vi "Set Fill Mode.vi"(8 "error in (no error)":errorcluster, 10 "Fill Mode":T1="ON", 11 "Instrument.1820 in":refnum<class "Instrument.Oxford1820.lvclass">) -> (0 "error out":errorcluster, 2 "Response":string, 3 "Instrument.1820 in":refnum<class "Instrument.Oxford1820.lvclass">)   [LabVIEW 2016, in "Instrument.Oxford1820.lvclass"]
uses:
  Instrument.Oxford1820.lvclass
  Typedefs/Fill Mode-Combo.ctl
  Typedefs/Instrument.Oxford1820.Commands-enum.ctl
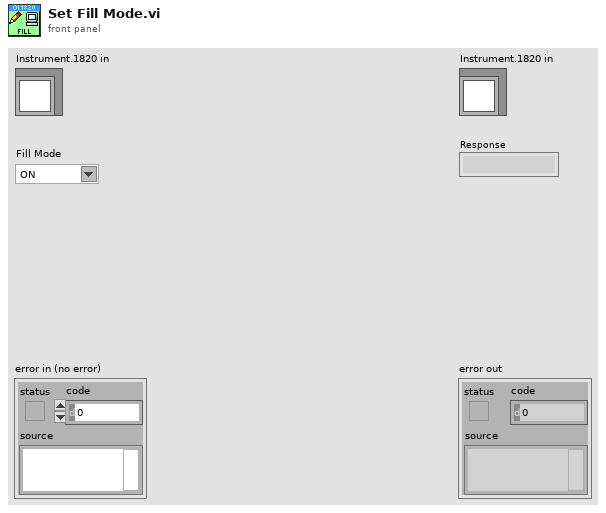
[diagram p1: front panel]
types:
  T1 = typedef "Instrument.Oxford1820.lvclass/Fill Mode-Combo.ctl" = string
  T2 = typedef "Instrument.Oxford1820.lvclass/Instrument.Oxford1820.Commands-enum.ctl" = enum16{"setAction", "setTarget", "setSwitchHeat", "setLambda", "setFillMode", "setNeedleValve", "setMagnetField", "getStatus", "getTarget", "getSwitchHeat", "getPSUField", "newcommand", "getMagnetField"}
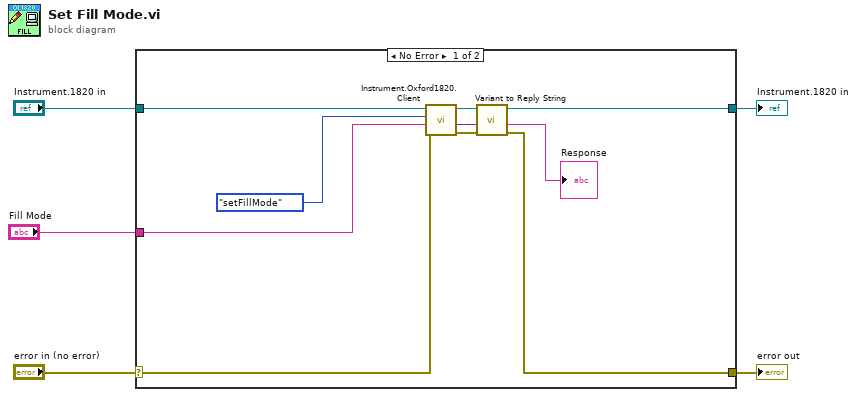
[diagram p0: block diagram]
diagram:
  n1 = case shown="No Error" "error in (no error)" {
    selector: "error in (no error)" -> [w14 w17]
    tunnel: [w8 w17] -> w4
    tunnel: [w6 w16] -> w2
    tunnel: "Instrument.1820 in" -> [w12 w16]
    tunnel: "Fill Mode" -> [w13 _]
    frame No Error {
      n2 = call "Instrument.Oxford1820.Client.vi"("error in (no error)"=w14, "Data"=w13, "Commands"=Instrument.Oxford1820.Commands-enum."setFillMode", "Instrument.1820 in"=w12) -> ("error out"=w9:errorcluster, "Data out"=w10:variant, "Instrument.1820 out"=w7:refnum<class "Instrument.Oxford1820.lvclass">)  [unwired: 5 in]
      n3 = call "Variant to Reply String.vi"("error in (no error)"=w9, "Data"=w10, "Instrument.1820 in"=w7) -> ("error out"=w8:errorcluster, "Reply"=→"Response":string, "Instrument.1820 out"=w6:refnum<class "Instrument.Oxford1820.lvclass">)  [unwired: 6 in]
    }
    frame Error {
    }
  }
  "error out" <- w4
  "Instrument.1820 in" <- w2
